vi "MGI Coerce Radians.vi"(1 "Radians":sgl format="%.2f") -> (0 "-pi to +pi":sgl format="%.2f")   [LabVIEW 2020]
doc: "Coerce an angle in radians to the range +/-pi.\n\nAuthored by David A. Moore\nsupport@mooregoodideas.com\nwww.mooregoodideas.com\n\nCopyright (c) 2010, Moore Good Ideas, Inc.\n\nAll rights reserved.\n\nRedistribution and use in source and binary forms, with or without modification, are permitted provided that the following conditions are met:\n\n * Redistributions of source code must retain the above copyright notice, this list of conditions and the following disclaimer.\n * Redistributions in binary form must reproduce the above copyright notice, this list of conditions and the following disclaimer in the documentation and/or other materials provided with the distribution.\n * Neither the name of Moore Good Ideas, Inc. nor the names of its contributors may be used to endorse or promote products derived from this software without specific prior written permission.\n\nTHIS SOFTWARE IS PROVIDED BY THE COPYRIGHT HOLDERS AND CONTRIBUTORS \"AS IS\" AND ANY EXPRESS OR IMPLIED WARRANTIES, INCLUDING, BUT NOT LIMITED TO, THE IMPLIED WARRANTIES OF MERCHANTABILITY AND FITNESS FOR A PARTICULAR PURPOSE ARE DISCLAIMED. IN NO EVENT SHALL THE COPYRIGHT OWNER OR CONTRIBUTORS BE LIABLE FOR ANY DIRECT, INDIRECT, INCIDENTAL, SPECIAL, EXEMPLARY, OR CONSEQUENTIAL DAMAGES (INCLUDING, BUT NOT LIMITED TO, PROCUREMENT OF SUBSTITUTE GOODS OR SERVICES; LOSS OF USE, DATA, OR PROFITS; OR BUSINESS INTERRUPTION) HOWEVER CAUSED AND ON ANY THEORY OF LIABILITY, WHETHER IN CONTRACT, STRICT LIABILITY, OR TORT (INCLUDING NEGLIGENCE OR OTHERWISE) ARISING IN ANY WAY OUT OF THE USE OF THIS SOFTWARE, EVEN IF ADVISED OF THE POSSIBILITY OF SUCH DAMAGE."
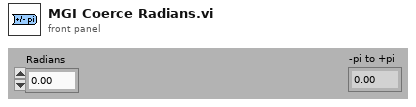
[diagram p1: front panel]
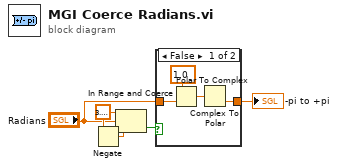
[diagram p0: block diagram]
diagram:
  w5 = sgl 3.1415927
  n1 = Negate(x=w5) -> (-x=w4:sgl)
  n2 = In Range and Coerce(upper limit=w5, x="Radians", lower limit=w4) -> (In Range?=w3:bool)  [unwired: 1 out]
  n3 = case shown="False" w3 {
    tunnel: "Radians" -> [w9 w10]
    tunnel: [w6 w10] -> w1
    frame False {
      n4 = Polar To Complex(1:w9, 2:sgl 1.0 ("r")) -> (0:w7:csg)
      n5 = Complex To Polar(r * e^(i*theta)=w7) -> (theta=w6:sgl)  [unwired: 1 out]
    }
    frame True {
    }
  }
  "-pi to +pi" <- w1
